vi "Teleop.vi"(10 "Match Info":T1={"Autonomous Elapsed Seconds"=0.0, "TeleOp Elapsed Seconds"=0.0, "Disabled Elapsed Seconds"=0.0, "Visited Autonomous"=FALSE, "Visited TeleOp"=FALSE, "Visited Disabled"=FALSE, "Autonomous Settings"={"Autonomous Style"=enum."Independent", "VI Refnum"=refnum}}, 11 "Call Context":T2) -> ()   [LabVIEW 2015]
doc: "This VI is called for each TeleOp packet received from the DS where the robot is not disabled. It is often used to read from the joysticks and update I/O or to update setpoints for timed control loops. It should complete and return within 20 milliseconds or it may miss DS packets."
uses:
  <vilib>/Rock Robotics/WPI/DriverStation/WPI_DriverStationDerivedRobotMode.ctl
  <vilib>/Rock Robotics/WPI/DriverStation/WPI_DriverStationMatch Info.ctl
  <vilib>/Rock Robotics/WPI/Utilities/WPI_GetSetVariantRefNum.vi
  <vilib>/Rock Robotics/Network Tables/NT Write Boolean Array.vi
  <vilib>/Rock Robotics/Network Tables/NT Write Numeric Array.vi
  <vilib>/Rock Robotics/Network Tables/NT Read Boolean.vi
  <vilib>/Rock Robotics/Network Tables/NT Read Number.vi
  <vilib>/Rock Robotics/Network Tables/NT Write Number.vi
  <vilib>/Rock Robotics/Network Tables/NT Write Boolean.vi
panel:
  out "Switch Pressed 2":bool
  out "Switch Pressed":bool
  out "Sample Slider 0":dbl(slide) scale=0.0..5.0
  out "Sample Boolean 1":bool
  out "Sample Boolean 0":bool
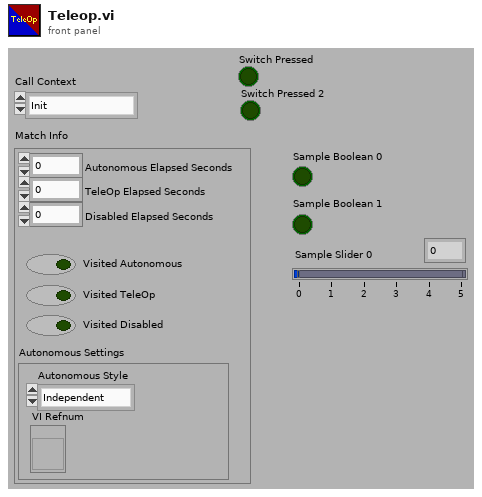
[diagram p1: front panel]
types:
  T1 = typedef "WPI_DriverStationMatch Info.ctl" = cluster{"Autonomous Elapsed Seconds":dbl, "TeleOp Elapsed Seconds":dbl, "Disabled Elapsed Seconds":dbl, "Visited Autonomous":bool, "Visited TeleOp":bool, "Visited Disabled":bool, "Autonomous Settings":cluster{"Autonomous Style":enum16{"Iterative", "Independent"}, "VI Refnum":refnum<vi>}}
  T2 = typedef "WPI_DriverStationDerivedRobotMode.ctl" = enum16{"Init", "Execute", "Stop"}
  T3 = typedef "WPI_JoystickDevRef.ctl" = cluster{"Device":T4}
  T4 = typedef "WPI_JoystickDeviceEnum.ctl" = enum16{"USB 0", "USB 1", "USB 2", "USB 3", "USB 4", "USB 5"}
  T5 = typedef "WPI_SwitchDevRef.ctl" = cluster{"DevStatus":errorcluster, "DIO Channel":T6, "CntIndex":T7, "Normally Closed":bool}
  T6 = typedef "FPGA_DIOChannel.ctl" = enum8{"DIO 0", "DIO 1", "DIO 2", "DIO 3", "DIO 4", "DIO 5", "DIO 6", "DIO 7", "DIO 8", "DIO 9", "DIO MXP 0", "DIO MXP 1", "DIO MXP 2", "DIO MXP 3", "DIO MXP 4", "DIO MXP 5", "DIO MXP 6", "DIO MXP 7", "DIO MXP 8", "DIO MXP 9", "DIO MXP 10", "DIO MXP 11", "DIO MXP 12", "DIO MXP 13", "DIO MXP 14", "DIO MXP 15", "Invalid"}
  T7 = typedef "FPGA_CounterCtrSystemIndex.ctl" = enum8{"Ctr 0", "Ctr 1", "Ctr 2", "Ctr 3", "Ctr 4", "Ctr 5", "Ctr 6", "Ctr 7", "Invalid"}
  T8 = typedef "WPI_EncoderDevRef.ctl" = cluster{"DevStatus":errorcluster, "EncoderIndex":T9, "CounterIndex":T7, "DistancePerCount":dbl, "Decoding Type":T10}
  T9 = typedef "FPGA_EncoderIdx.ctl" = enum8{"Enc 0", "Enc 1", "Enc 2", "Enc 3", "Enc 4", "Enc 5", "Enc 6", "Enc 7", "Invalid"}
  T10 = typedef "WPI_EncoderType.ctl" = enum16{"1x", "2x", "4x"}
  T11 = typedef "WPI_RobotDriveDevRef.ctl" = cluster{"DevStatus":errorcluster, "Motors[]":T12[], "Square Inputs":bool, "Max Output":dbl}
  T12 = typedef "WPI_MotorControlDeviceRef.ctl" = cluster{"DeviceStatus":errorcluster, "Type":T13, "PWM":cluster{"PWM Channel":T14, "DeadBand":T15}, "CAN":cluster{"Device Number":u8, "Control Mode":T16, "Semaphore":T17, "Max Vout":dbl, "TalonSRX Control Mode":T18}, "Invert":bool}
  T13 = typedef "WPI_MotorControlType.ctl" = enum16{"PWM", "CAN", "CANTalonSRX"}
  T14 = typedef "FPGA_DIOPWMChannel.ctl" = enum8{"PWM 0", "PWM 1", "PWM 2", "PWM 3", "PWM 4", "PWM 5", "PWM 6", "PWM 7", "PWM 8", "PWM 9", "PWM MXP 0", "PWM MXP 1", "PWM MXP 2", "PWM MXP 3", "PWM MXP 4", "PWM MXP 5", "PWM MXP 6", "PWM MXP 7", "PWM MXP 8", "PWM MXP 9", "Invalid"}
  T15 = typedef "WPI_PWMDeadband.ctl" = cluster{"Name":string, "maxPositivePwm":i32, "minPositivePwm":i32, "centerPwm":i32, "maxNegativePwm":i32, "minNegativePwm":i32, "angularRange":u16}
  T16 = typedef "WPI_CANJaguar_ControlMode.ctl" = enum8{"Percent VBus", "Current", "Speed", "Position", "Voltage"}
  T17 = typedef "Semaphore RefNum" = refnum<k1>
  T18 = typedef "WPI_CANTalonSRX_APIControlMode.ctl" = enum8{"Percent VBus", "Speed", "Position", "Slave", "Unchanged / Invalid", "Voltage Compensation", "Current", "Motion Profile"}
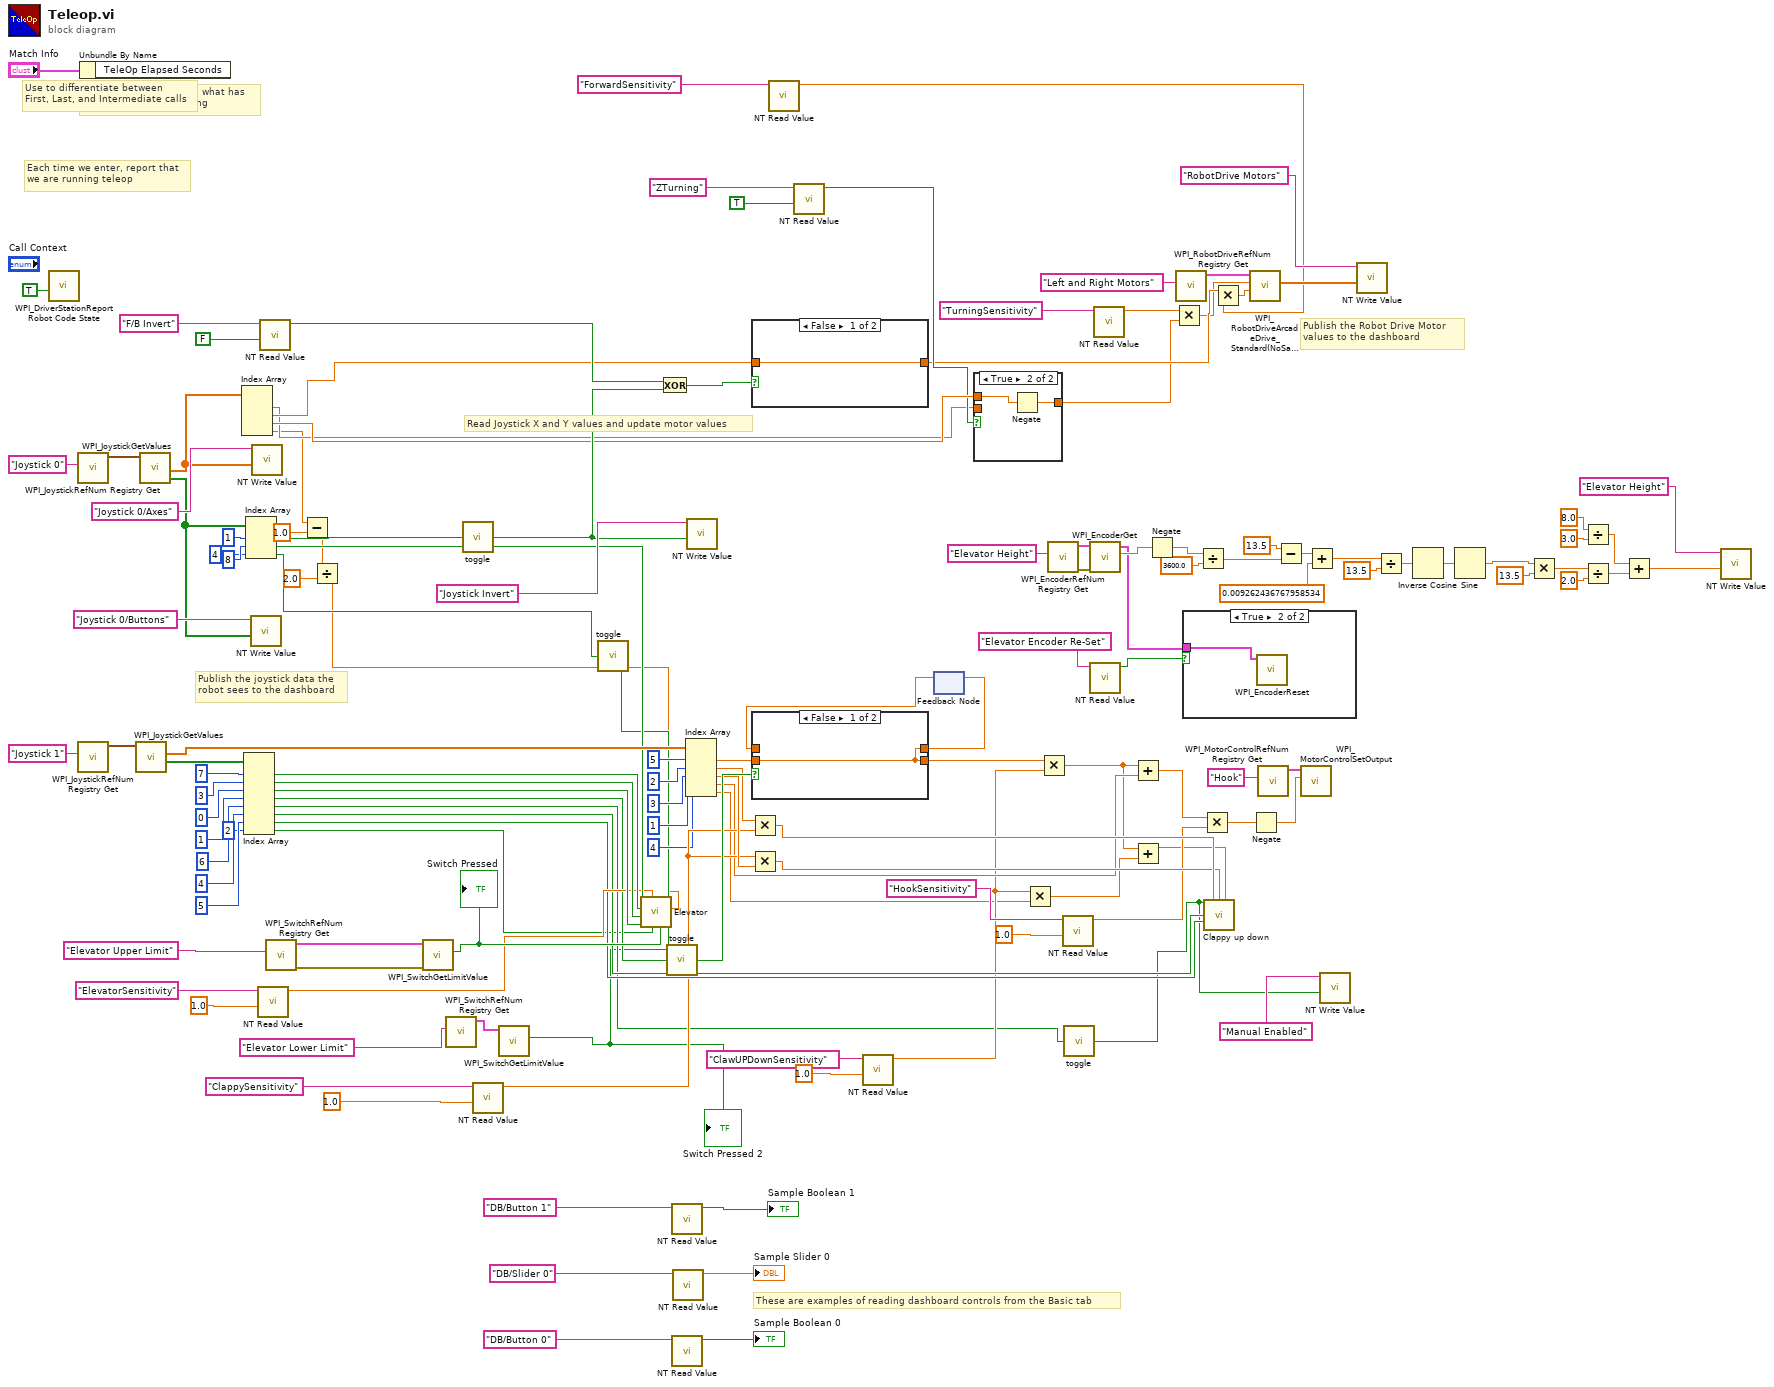
[diagram p0: block diagram]
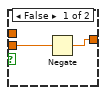
[diagram p4: hidden frame]
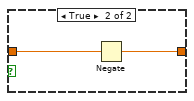
[diagram p5: hidden frame]
diagram:
  # "These are examples of reading dashboard controls from the Basic tab"
  # "Publish the Robot Drive Motor\nvalues to the dashboard"
  # "Publish the joystick data the\nrobot sees to the dashboard"
  # "Each time we enter, report that\nwe are running teleop"
  # "Use to differentiate between\nFirst, Last, and Intermediate calls"
  # "This can help determine what has\nbeen run and for how long"
  # "Read Joystick X and Y values and update motor values"
  n1 = call <vilib>:"WPI_DriverStationReport Robot Code State.vi"("TeleOp"=TRUE ("Autonomous")) -> ()  [unwired: 10 in, 1 out]
  n2 = call <vilib>:"WPI_JoystickRefNum Registry Get.vi"("refnum name"="Joystick 0") -> ("JoystickDevRef"=w138:T3)  [unwired: 1 in, 9 out]
  n3 = call <vilib>:"WPI_JoystickRefNum Registry Get.vi"("refnum name"="Joystick 1") -> ("JoystickDevRef"=w111:T3)  [unwired: 1 in, 9 out]
  n4 = Unbundle By Name("Match Info") -> ()  [unwired: 1 out]
  n5 = call <vilib>:"WPI_JoystickGetValues.vi"("JoystickDevRef"=w111) -> ("Buttons"=w103:bool[], "Axes"=w110:dbl[])  [unwired: 6 in, 3 out]
  n6 = call <vilib>:"WPI_JoystickGetValues.vi"("JoystickDevRef"=w138) -> ("Buttons"=w120:bool[], "Axes"=w134:dbl[])  [unwired: 6 in, 3 out]
  n7 = Index Array(array=w134) -> (element #1=w49:dbl, element #2=w50:dbl, element #3=w116:dbl, element #4=w38:dbl)  [unwired: 4 in]
  n8 = Index Array(array=w103, index #1=7 ("index"), index #2=3 ("index"), index #3=0 ("index"), index #4=1 ("index"), index #5=6 ("index"), index #6=4 ("index"), index #7=5 ("index"), index #8=2 ("index")) -> (element #1=w101:bool, element #2=w100:bool, element #3=w98:bool, element #4=w87:bool, element #5=w52:bool, element #6=w81:bool, element #7=w80:bool, element #8=w39:bool)
  n9 = Index Array(array=w120, index #1=1 ("index"), index #2=8 ("index"), index #3=4 ("index")) -> (element #1=w118:bool, element #2=w104:bool, element #3=w42:bool)
  n10 = call-poly <vilib>:"NT Write Value.vi"("Boolean Array"=w120, "Name"="Joystick 0/Buttons") -> ()  [unwired: 9 in, 1 out]
  n11 = call-poly <vilib>:"NT Write Value.vi"("Numeric Array"=w134, "Name"="Joystick 0/Axes") -> ()  [unwired: 9 in, 1 out]
  n12 = call-poly <vilib>:"NT Read Value.vi"("Default Value"=1.0, "Name"="ElevatorSensitivity") -> ("Numeric"=w95:dbl)  [unwired: 8 in, 1 out]
  n13 = call-poly <vilib>:"NT Read Value.vi"("Default Value"=FALSE, "Name"="F/B Invert") -> ("Boolean"=w123:bool)  [unwired: 8 in, 1 out]
  n14 = call <vilib>:"WPI_SwitchRefNum Registry Get.vi"("refnum name"="Elevator Upper Limit") -> ("error out"=w109:errorcluster, "SwitchDevRef"=w108:T5)  [unwired: 9 in]
  n15 = Subtract(x=w38, y=1.0) -> (x-y=w37:dbl)
  n16 = Divide(x=w37, y=2.0) -> (x/y=w35:dbl)
  n17 = call <vilib>:"WPI_SwitchGetLimitValue.vi"("error in (no error)"=w109, "SwitchDevRef"=w108) -> ("Switch Pressed"=w106:bool)  [unwired: 7 in, 2 out]
  "Switch Pressed" <- w106
  n18 = call <vilib>:"WPI_SwitchRefNum Registry Get.vi"("refnum name"="Elevator Lower Limit") -> ("SwitchDevRef"=w45:T5)  [unwired: 9 in, 1 out]
  n19 = call "toggle.vi"("Input"=w118) -> ("Output"=w117:bool)
  n20 = call-poly <vilib>:"NT Read Value.vi"("Default Value"=1.0, "Name"="ClappySensitivity") -> ("Numeric"=w73:dbl)  [unwired: 8 in, 1 out]
  n21 = call <vilib>:"WPI_SwitchGetLimitValue.vi"("SwitchDevRef"=w45) -> ("Switch Pressed"=w44:bool)  [unwired: 8 in, 2 out]
  "Switch Pressed 2" <- w44
  n22 = call "toggle.vi"("Input"=w42) -> ("Output"=w41:bool)
  n23 = call "Elevator.vi"("Lower Limit Switch"=w44, "Driver Elevator Speed"=w35, "Driver Invert"=w41, "Upper Limit Switch"=w106, "Give Driver Control?"=w39, "ELEV SEMSITIVITY"=w95, "Lower"=w98, "Raise"=w100, "Override CoPilot"=w101, "Override Pilot"=w104) -> ()  [unwired: 1 in]
  n24 = Exclusive Or(1:w117, 2:w123) -> (0:w122:bool)
  n25 = call "toggle.vi"("Input"=w87) -> ("Output"=w90:bool)
  n26 = call-poly <vilib>:"NT Read Value.vi"("Name"="DB/Button 1" ("refnum name")) -> ("Boolean"=→"Sample Boolean 1":bool)  [unwired: 9 in, 1 out]
  n27 = call-poly <vilib>:"NT Read Value.vi"("Name"="DB/Button 0" ("refnum name")) -> ("Boolean"=→"Sample Boolean 0":bool)  [unwired: 9 in, 1 out]
  n28 = call-poly <vilib>:"NT Read Value.vi"("Name"="DB/Slider 0" ("refnum name")) -> ("Numeric"=→"Sample Slider 0":dbl)  [unwired: 9 in, 1 out]
  n29 = Index Array(array=w110, index #1=5 ("index"), index #2=2 ("index"), index #3=3 ("index"), index #4=1 ("index"), index #5=4 ("index")) -> (element #1=w94:dbl, element #2=w84:dbl, element #3=w83:dbl, element #4=w61:dbl, element #5=w54:dbl)
  n30 = call-poly <vilib>:"NT Write Value.vi"("Boolean"=w117, "Name"="Joystick Invert") -> ()  [unwired: 9 in, 1 out]
  n31 = Multiply(x=w84, y=w73) -> (x*y=w75:dbl)
  n32 = Multiply(x=w73, y=w83) -> (x*y=w74:dbl)
  n33 = case shown="False" w122 {
    tunnel: [w143 w144] -> w48
    tunnel: w50 -> [w143 w145]
    frame False {
    }
    frame True {
      n34 = Negate(x=w145) -> (-x=w144:dbl)
    }
  }
  n35 = call-poly <vilib>:"NT Read Value.vi"("Name"="ForwardSensitivity") -> ("Numeric"=w2:dbl)  [unwired: 9 in, 1 out]
  n36 = call-poly <vilib>:"NT Read Value.vi"("Default Value"=TRUE, "Name"="ZTurning") -> ("Boolean"=w113:bool)  [unwired: 8 in, 1 out]
  n37 = call-poly <vilib>:"NT Read Value.vi"("Default Value"=1.0, "Name"="ClawUPDownSensitivity") -> ("Numeric"=w55:dbl)  [unwired: 8 in, 1 out]
  n38 = feedback #1() -> (w92:dbl)  [unwired: 1 in]
  n39 = case shown="False" w90 {
    tunnel: [w146 w147] -> w91
    tunnel: w94 -> [w146 _]
    tunnel: [w146 w147] -> w64
    tunnel: w92 -> [_ w147]
    frame False {
    }
    frame True {
    }
  }
  n40 = feedback-in #1(w91) -> ()
  n41 = case shown="True" w113 {
    tunnel: w116 -> [_ w151]
    tunnel: w49 -> [w149 _]
    tunnel: [w148 w150] -> w47
    frame False {
      n42 = Negate(x=w149) -> (-x=w148:dbl)
    }
    frame True {
      n43 = Negate(x=w151) -> (-x=w150:dbl)
    }
  }
  n44 = Multiply(x=w55, y=w54) -> (x*y=w56:dbl)
  n45 = Multiply(x=w64, y=w55) -> (x*y=w59:dbl)
  n46 = call <vilib>:"WPI_EncoderRefNum Registry Get.vi"("refnum name"="Elevator Height") -> ("error out"=w32:errorcluster, "EncoderDevRef"=w31:T8)  [unwired: 9 in]
  n47 = call-poly <vilib>:"NT Read Value.vi"("Default Value"=1.0, "Name"="HookSensitivity") -> ("Numeric"=w60:dbl)  [unwired: 8 in, 1 out]
  n48 = call "toggle.vi"("Input"=w52) -> ("Output"=w51:bool)
  n49 = call <vilib>:"WPI_EncoderGet.vi"("error in (no error)"=w32, "EncoderDevRef"=w31) -> ("Distance"=w20:dbl, "EncoderDevRef"=w14:T8)  [unwired: 4 in, 4 out]
  n50 = call-poly <vilib>:"NT Read Value.vi"("Name"="Elevator Encoder Re-Set") -> ("Boolean"=w13:bool)  [unwired: 9 in, 1 out]
  n51 = call-poly <vilib>:"NT Read Value.vi"("Name"="TurningSensitivity") -> ("Numeric"=w4:dbl)  [unwired: 9 in, 1 out]
  n52 = Add(x=w59, y=w61) -> (x+y=w67:dbl)
  n53 = Add(x=w59, y=w56) -> (x+y=w57:dbl)
  n54 = Negate(x=w20) -> (-x=w11:dbl)
  n55 = Multiply(x=w4, y=w47) -> (x*y=w6:dbl)
  n56 = call <vilib>:"WPI_RobotDriveRefNum Registry Get.vi"("refnum name"="Left and Right Motors") -> ("RobotDriveDevRef"=w140:T11)  [unwired: 1 in, 9 out]
  n57 = case shown="True" w13 {
    tunnel: w14 -> [_ w152]
    frame False {
    }
    frame True {
      n58 = call <vilib>:"WPI_EncoderReset.vi"("EncoderDevRef"=w152) -> ()  [unwired: 9 in, 2 out]
    }
  }
  n59 = Divide(x=w11, y=3600.0 ("x")) -> (x/y=w25:dbl)
  n60 = Multiply(x=w67, y=w60) -> (x*y=w63:dbl)
  n61 = call "Clappy up down.vi"("Manual"=w51, "Open/Closed 1"=w75, "Open/Closed 2"=w74, "UP/Down"=w57, "Negate 1"=w81, "Negate 2"=w80) -> ()  [unwired: 10 in]
  n62 = Multiply(x=w48, y=w2) -> (x*y=w1:dbl)
  n63 = call <vilib>:"WPI_RobotDriveArcadeDrive_Standard(NoSaturation).vi"("Y axis value"=w1, "X axis value"=w6, "RobotDriveDevRef"=w140) -> ("Motor Values"=w127:dbl[])  [unwired: 1 in, 7 out]
  n64 = Negate(x=w63) -> (-x=w68:dbl)
  n65 = call <vilib>:"WPI_MotorControlRefNum Registry Get.vi"("refnum name"="Hook") -> ("MotorControlDevRef"=w71:T12)  [unwired: 9 in, 1 out]
  n66 = Subtract(x=13.5, y=w25) -> (x-y=w23:dbl)
  n67 = call <vilib>:"WPI_MotorControlSetOutput.vi"("Output"=w68, "MotorControlDevRef"=w71) -> ()  [unwired: 7 in, 3 out]
  n68 = Add(x=w23, y=0.009262436767958534) -> (x+y=w22:dbl)
  n69 = call-poly <vilib>:"NT Write Value.vi"("Boolean"=w51, "Name"="Manual Enabled") -> ()  [unwired: 9 in, 1 out]
  n70 = call-poly <vilib>:"NT Write Value.vi"("Numeric Array"=w127, "Name"="RobotDrive Motors") -> ()  [unwired: 9 in, 1 out]
  n71 = Divide(x=w22, y=13.5) -> (x/y=w29:dbl)
  n72 = Inverse Cosine(1:w29) -> (0:w28:dbl)
  n73 = Sine(x=w28) -> (sin(x)=w27:dbl)
  n74 = Multiply(x=w27, y=13.5) -> (x*y=w15:dbl)
  n75 = Divide(x=8.0, y=3.0) -> (x/y=w7:dbl)
  n76 = Divide(x=w15, y=2.0) -> (x/y=w18:dbl)
  n77 = Add(x=w7, y=w18) -> (x+y=w10:dbl)
  n78 = call-poly <vilib>:"NT Write Value.vi"("Numeric"=w10, "Name"="Elevator Height") -> ()  [unwired: 9 in, 1 out]
